vi "VI Tree.vi"   [LabVIEW 2015, in "Tektronix 7000 Series.lvlib"]
doc: "This VI displays all the instrument driver VIs for the Tektronix TDS5k Series,TDS6k Series,TDS7k Series, DPO7k Series, DPO70k Series, DSA70k Series, MSO5k Series, DPO5k Series oscilloscopes. The block diagram window displays all the user-callable VIs of the instrument driver in an organized table."
uses:
  <instrlib>/Tektronix 7000 Series/Tektronix 7000 Series.lvlib
  <instrlib>/Tektronix 7000 Series/Public/Data/Low Level/Fetch Waveform Measurement (More).vi
  <instrlib>/Tektronix 7000 Series/Public/Data/Low Level/Fetch (Waveform).vi
  <instrlib>/Tektronix 7000 Series/Public/Configure/Math/Configure Math Expression (Unary Operation).vi
  <instrlib>/Tektronix 7000 Series/Public/Configure/Math/Configure Spectral (Magnitude).vi
  <instrlib>/Tektronix 7000 Series/Public/Configure/Math/Configure Math (Basic).vi
  <instrlib>/Tektronix 7000 Series/Public/Configure/Configure Bus Source (I2C).vi
  <instrlib>/Tektronix 7000 Series/Public/Configure/Configure Trigger (A Mode).vi
  <instrlib>/Tektronix 7000 Series/Public/Data/Read (Single Waveform).vi
  <instrlib>/Tektronix 7000 Series/Public/Data/Read Waveform Measurement (Amplitude).vi
panel:
  # "Copyright 2006 - 2016 National Instruments Corporation.  ALL RIGHTS RESERVED."
  # "SEE DIAGRAM\nFOR VI TREE."
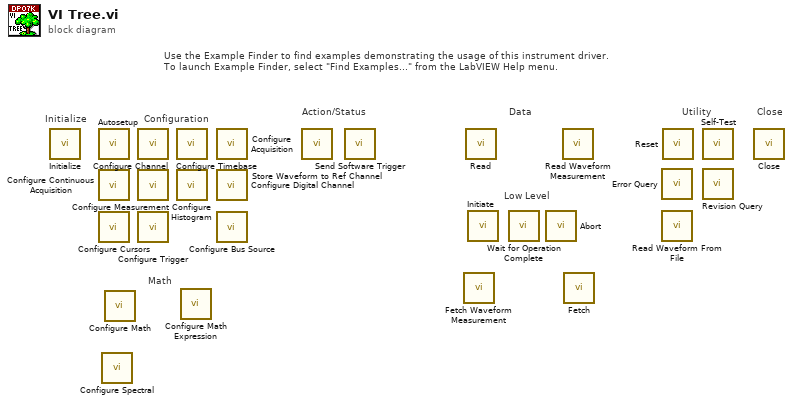
[diagram p0: block diagram]
diagram:
  # "Use the Example Finder to find examples demonstrating the usage of this instrument driver.\nTo launch Example Finder, select \"Find Examples...\" from the LabVIEW Help menu."
  # "Math"
  # "Low Level"
  # "Action/Status"
  # "Configuration"
  # "Utility"
  # "Data"
  # "Close"
  # "Initialize"
  n1 = call <instrlib>:"Initialize.vi"() -> ()  [unwired: 10 in, 2 out]
  n2 = call <instrlib>:"Autosetup.vi"() -> ()  [unwired: 10 in, 2 out]
  n3 = call <instrlib>:"Configure Continuous Acquisition.vi"() -> ()  [unwired: 10 in, 2 out]
  n4 = call <instrlib>:"Configure Cursors.vi"() -> ()  [unwired: 14 in, 2 out]
  n5 = call-poly <instrlib>:"Configure Spectral.vi"() -> ()  [unwired: 14 in, 2 out]
  n6 = call-poly <instrlib>:"Configure Math.vi"() -> ()  [unwired: 10 in, 2 out]
  n7 = call <instrlib>:"Configure Channel.vi"() -> ()  [unwired: 14 in, 2 out]
  n8 = call <instrlib>:"Configure Measurement.vi"() -> ()  [unwired: 14 in, 2 out]
  n9 = call-poly <instrlib>:"Configure Trigger.vi"() -> ()  [unwired: 14 in, 2 out]
  n10 = call <instrlib>:"Configure Timebase.vi"() -> ()  [unwired: 10 in, 2 out]
  n11 = call <instrlib>:"Configure Histogram.vi"() -> ()  [unwired: 14 in, 2 out]
  n12 = call-poly <instrlib>:"Configure Math Expression.vi"() -> ()  [unwired: 9 in, 3 out]
  n13 = call <instrlib>:"Configure Acquisition.vi"() -> ()  [unwired: 14 in, 2 out]
  n14 = call <instrlib>:"Configure Digital Channel.vi"() -> ()  [unwired: 10 in, 2 out]
  n15 = call-poly <instrlib>:"Configure Bus Source.vi"() -> ()  [unwired: 10 in, 2 out]
  n16 = call <instrlib>:"Store Waveform to Ref Channel.vi"() -> ()  [unwired: 10 in, 2 out]
  n17 = call <instrlib>:"Send Software Trigger.vi"() -> ()  [unwired: 10 in, 2 out]
  n18 = call-poly <instrlib>:"Fetch Waveform Measurement.vi"() -> ()  [unwired: 13 in, 3 out]
  n19 = call-poly <instrlib>:"Read.vi"() -> ()  [unwired: 9 in, 3 out]
  n20 = call <instrlib>:"Initiate.vi"() -> ()  [unwired: 10 in, 2 out]
  n21 = call <instrlib>:"Wait for Operation Complete.vi"() -> ()  [unwired: 10 in, 2 out]
  n22 = call <instrlib>:"Abort.vi"() -> ()  [unwired: 10 in, 2 out]
  n23 = call-poly <instrlib>:"Read Waveform Measurement.vi"() -> ()  [unwired: 13 in, 3 out]
  n24 = call-poly <instrlib>:"Fetch.vi"() -> ()  [unwired: 9 in, 3 out]
  n25 = call <instrlib>:"Error Query.vi"() -> ()  [unwired: 8 in, 4 out]
  n26 = call <instrlib>:"Read Waveform From File.vi"() -> ()  [unwired: 10 in, 6 out]
  n27 = call <instrlib>:"Reset.vi"() -> ()  [unwired: 10 in, 2 out]
  n28 = call <instrlib>:"Self-Test.vi"() -> ()  [unwired: 8 in, 4 out]
  n29 = call <instrlib>:"Revision Query.vi"() -> ()  [unwired: 8 in, 4 out]
  n30 = call <instrlib>:"Close.vi"() -> ()  [unwired: 11 in, 1 out]
